vi "Write.vi"(8 "error in (no error)":errorcluster, 11 "RT Data in":T1 {"Channels"."Voltage"."Ref"."Data Reference" format="%.0x"; "Channels"."Current"."Ref"."Data Reference" format="%.0x"; "Channels"."Read Volt"."Ref" format="%.0x"; "Channels"."Mode"."Ref" format="%.0x"}) -> (0 "error out":errorcluster, 3 "RT Data out":T1 {"Channels"."Voltage"."Ref"."Data Reference" format="%.0x"; "Channels"."Current"."Ref"."Data Reference" format="%.0x"; "Channels"."Read Volt"."Ref" format="%.0x"; "Channels"."Mode"."Ref" format="%.0x"})   [LabVIEW 2011, in "Switch-DMM Custom Device.lvlib"]
uses:
  Switch-DMM Custom Device.lvlib
  Controls/RT Data.ctl
  Controls/Channels.ctl
  Controls/Single Channel.ctl
  <vilib>/NI Veristand/Custom Device API/Data Reference.ctl
  Controls/Block Channels.ctl
  <vilib>/NI Veristand/Custom Device API/Block Data Reference.ctl
  Controls/Communication.ctl
  Controls/Async Status.ctl
  Controls/Async State.ctl
  Controls/Async Command.ctl
  Controls/Async Events.ctl
  <vilib>/NI Veristand/Custom Device API/Custom Device API.lvlib
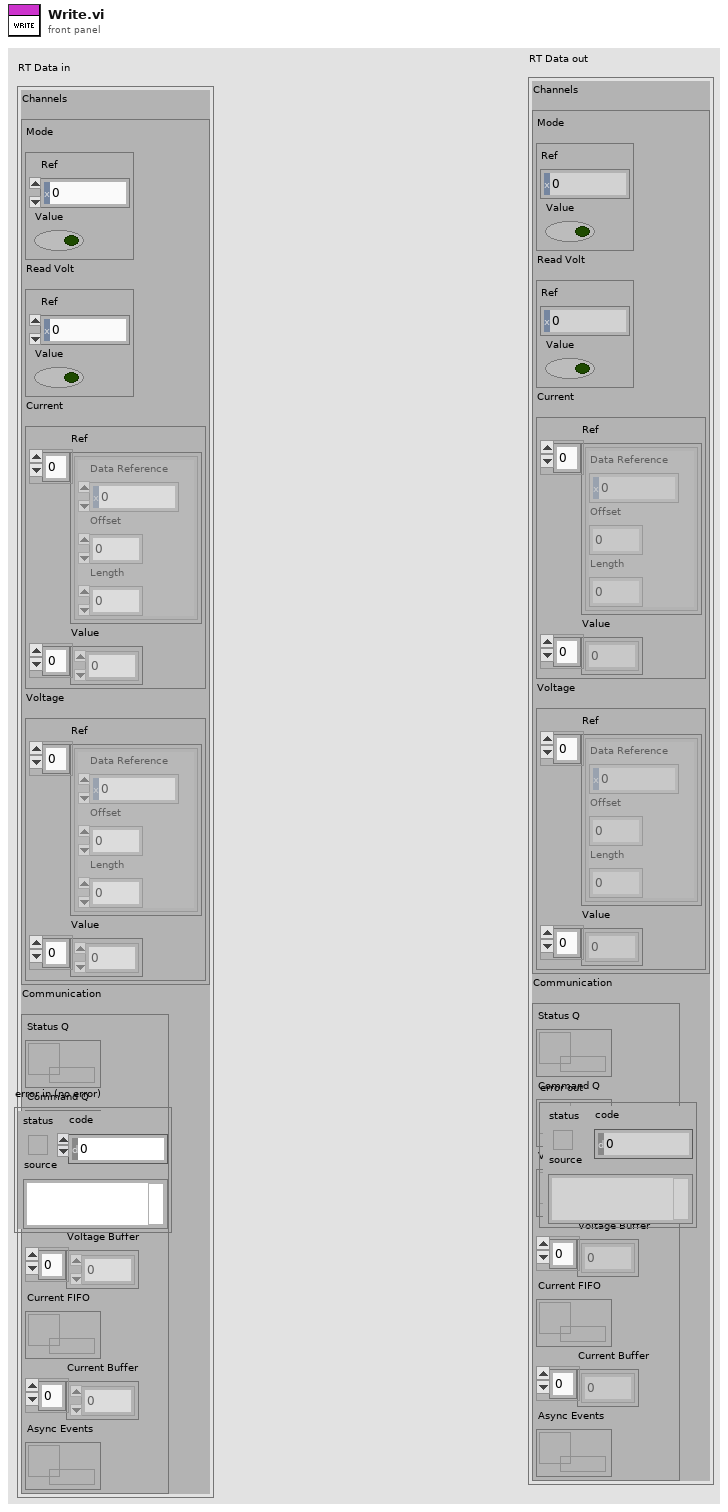
[diagram p1: front panel]
types:
  T1 = typedef "Switch-DMM Custom Device.lvlib/RT Data.ctl" = cluster{"Channels":T2, "Communication":T7}
  T2 = typedef "Switch-DMM Custom Device.lvlib/Channels.ctl" = cluster{"Mode":T3, "Read Volt":T3, "Current":T5, "Voltage":T5}
  T3 = typedef "Switch-DMM Custom Device.lvlib/Single Channel.ctl" = cluster{"Ref":T4, "Value":bool}
  T4 = typedef "Custom Device API.lvlib/Data Reference.ctl" = i32
  T5 = typedef "Switch-DMM Custom Device.lvlib/Block Channels.ctl" = cluster{"Ref":T6[], "Value":dbl[]}
  T6 = typedef "Custom Device API.lvlib/Block Data Reference.ctl" = cluster{"Data Reference":T4, "Offset":i32, "Length":i32}
  T7 = typedef "Switch-DMM Custom Device.lvlib/Communication.ctl" = cluster{"Status Q":refnum<queue>, "Command Q":refnum<queue>, "Voltage FIFO":refnum<k33>, "Voltage Buffer":dbl[], "Current FIFO":refnum<k33>, "Current Buffer":dbl[], "Async Events":refnum<queue>}
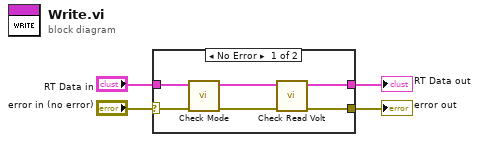
[diagram p0: block diagram]
diagram:
  n1 = case shown="No Error" "error in (no error)" {
    selector: "error in (no error)" -> [w9 w11]
    tunnel: "RT Data in" -> [w10 w12]
    tunnel: [w6 w12] -> w3
    tunnel: [w5 w11] -> w2
    frame No Error {
      n2 = call "Check Mode.vi"("error in (no error)"=w9, "RT Data in in"=w10) -> ("error out"=w7:errorcluster, "RT Data out"=w8:T1)  [unwired: 8 in]
      n3 = call "Check Read Volt.vi"("error in (no error)"=w7, "RT Data in in"=w8) -> ("error out"=w5:errorcluster, "RT Data out"=w6:T1)  [unwired: 8 in]
    }
    frame Error {
    }
  }
  "RT Data out" <- w3
  "error out" <- w2
